vi "P9374A NA setsweep.vi"(6 "Avg":i32=1, 7 "points":i32=1, 8 "error in (no error)":errorcluster {"code" format="%.0x"}, 11 "instrument handle":refnum<k15>) -> (0 "error out":errorcluster {"code" format="%.0x"}, 3 "instrument handle out":refnum<k15>)   [LabVIEW 2021]
uses:
  <instrlib>/Agilent NA/Agilent NA.lvlib
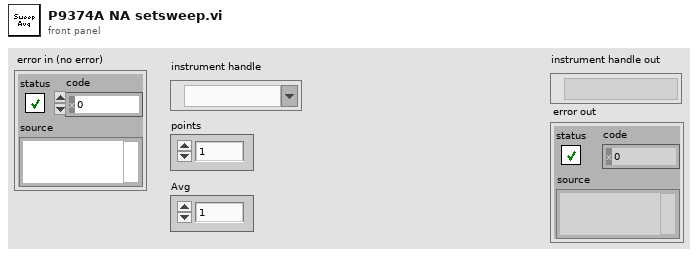
[diagram p1: front panel]
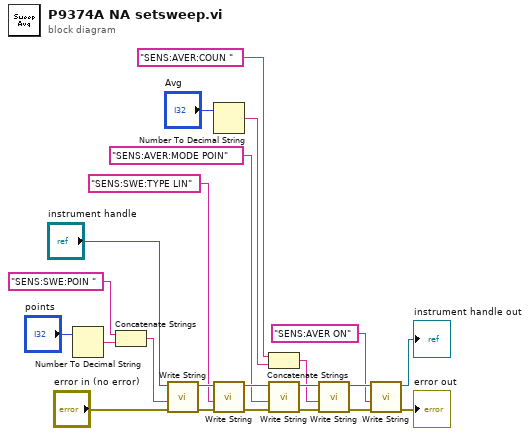
[diagram p0: block diagram]
diagram:
  n1 = Number To Decimal String(number="points") -> (decimal integer string=w20:string)  [unwired: 1 in]
  n2 = Concatenate Strings("SENS:SWE:POIN " ("string"), w20) -> (w18:string)
  n3 = call <instrlib>:"Write String.vi"("error in (no error)"="error in (no error)", "Command"=w18, "instrument handle"="instrument handle") -> ("error out"=w16:errorcluster, "instrument handle out"=w17:refnum<k15>)  [unwired: 7 in]
  n4 = Number To Decimal String(number="Avg") -> (decimal integer string=w7:string)  [unwired: 1 in]
  n5 = call <instrlib>:"Write String.vi"("error in (no error)"=w16, "Command"="SENS:SWE:TYPE LIN", "instrument handle"=w17) -> ("error out"=w13:errorcluster, "instrument handle out"=w14:refnum<k15>)  [unwired: 7 in]
  n6 = Concatenate Strings("SENS:AVER:COUN " ("string"), w7) -> (w6:string)
  n7 = call <instrlib>:"Write String.vi"("error in (no error)"=w13, "Command"="SENS:AVER:MODE POIN" ("string"), "instrument handle"=w14) -> ("error out"=w10:errorcluster, "instrument handle out"=w11:refnum<k15>)  [unwired: 7 in]
  n8 = call <instrlib>:"Write String.vi"("error in (no error)"=w10, "Command"=w6, "instrument handle"=w11) -> ("error out"=w4:errorcluster, "instrument handle out"=w5:refnum<k15>)  [unwired: 7 in]
  n9 = call <instrlib>:"Write String.vi"("error in (no error)"=w4, "Command"="SENS:AVER ON", "instrument handle"=w5) -> ("error out"=→"error out":errorcluster, "instrument handle out"=→"instrument handle out":refnum<k15>)  [unwired: 7 in]
